vi "_create_attribute_error.vi"(1 "Is Warning (False)":bool, 4 "Original error splitter (\"Original error:\")":string="\nOriginal error:\n", 5 "Error Elaboration (\"\")":string, 6 "Error creation enabled (T)":bool=TRUE, 7 "Attribute":T2={"Identifier"="", "Descriptive Name"="", "Data Type"=enum."Integer 32", "Command"="", "Access"=enum."Read/Write", "Range Table"="", "Read Callback"="", "Write Callback"="", "Supported Models"="", "Instrument Options"="", "Index"=0, "OPC Wait"=FALSE, "No Status Check"=FALSE, "Cache Only"=FALSE}, 8 "error in":errorcluster caption="error in (no error)", 9 "Additional detail from error source (\"\")":string, 10 "Error Enum in":T1=enum."VISA_err_Timeout", 11 "VISA resource name":refnum<visa-resource-name>) -> (0 "error out":errorcluster, 3 "VISA resource name out":refnum<visa-resource-name>)   [LabVIEW 2022 SP3, in "hmp4000_rsidr_core.lvlib"]
uses:
  hmp4000_rsidr_core.lvlib
  type_Attribute.ctl
  type_Attribute_Data_Type.ctl
  type_ReadWriteAccess.ctl
  type_Error_Codes.ctl
  Trim Whitespace One-Sided.vi
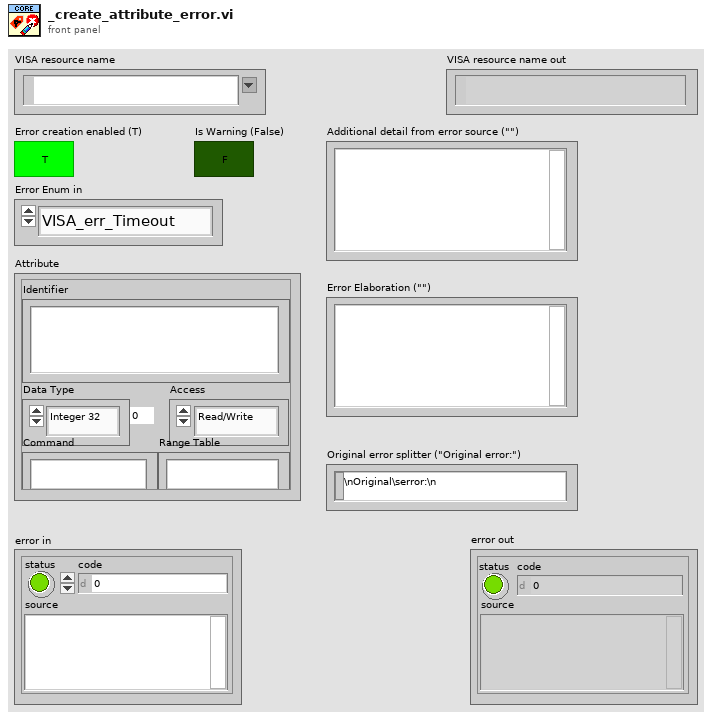
[diagram p1: front panel]
types:
  T1 = typedef "hmp4000_rsidr_core.lvlib/type_Error_Codes.ctl" = enum16{"No_error", "VISA_err_ResourceNotFound", "VISA_err_Timeout", "VISA_warn_MoreDataAvailable", "RS_err_MissingCallback", "RS_err_InvalidAttribute", "RS_err_InvalidValue", "RS_err_UnknownResource", "RS_err_AlreadyInitialized", "RS_err_InstrumentStatus", "RS_err_BadRepCapName", "RS_err_TypesMismatch", "RS_err_ValueNotSupported", "RS_err_InvalidRngTable", "RS_err_IDqueryFail", "RS_err_UnexpResponse", "VISA_warn_ConfigNotLoaded", "RS_err_AttributeNotReadable", "RS_err_AttributeNotWritable", "RS_err_InstrumentType", "RS_err_InstrumentOption", "VISA_err_InvalidSize", "RS_err_ReliabilityIndicator", "VISA_warn_UnknownStatus", "VISA_warn_TermCharRead", "VISA_err_IO_error", "RS_err_FunctionNotSupported", "VISA_warn_QueueEmpty"}
  T2 = typedef "hmp4000_rsidr_core.lvlib/type_Attribute.ctl" = cluster{"Identifier":string, "Descriptive Name":string, "Data Type":T3, "Command":string, "Access":T4, "Range Table":string, "Read Callback":string, "Write Callback":string, "Supported Models":string, "Instrument Options":string, "Index":i32, "OPC Wait":bool, "No Status Check":bool, "Cache Only":bool}
  T3 = typedef "hmp4000_rsidr_core.lvlib/type_Attribute_Data_Type.ctl" = enum16{"Integer 32", "Double", "String", "Boolean", "None", "Integer 64", "RawString"}
  T4 = typedef "hmp4000_rsidr_core.lvlib/type_ReadWriteAccess.ctl" = enum16{"Read Only", "Write Only", "Read/Write"}
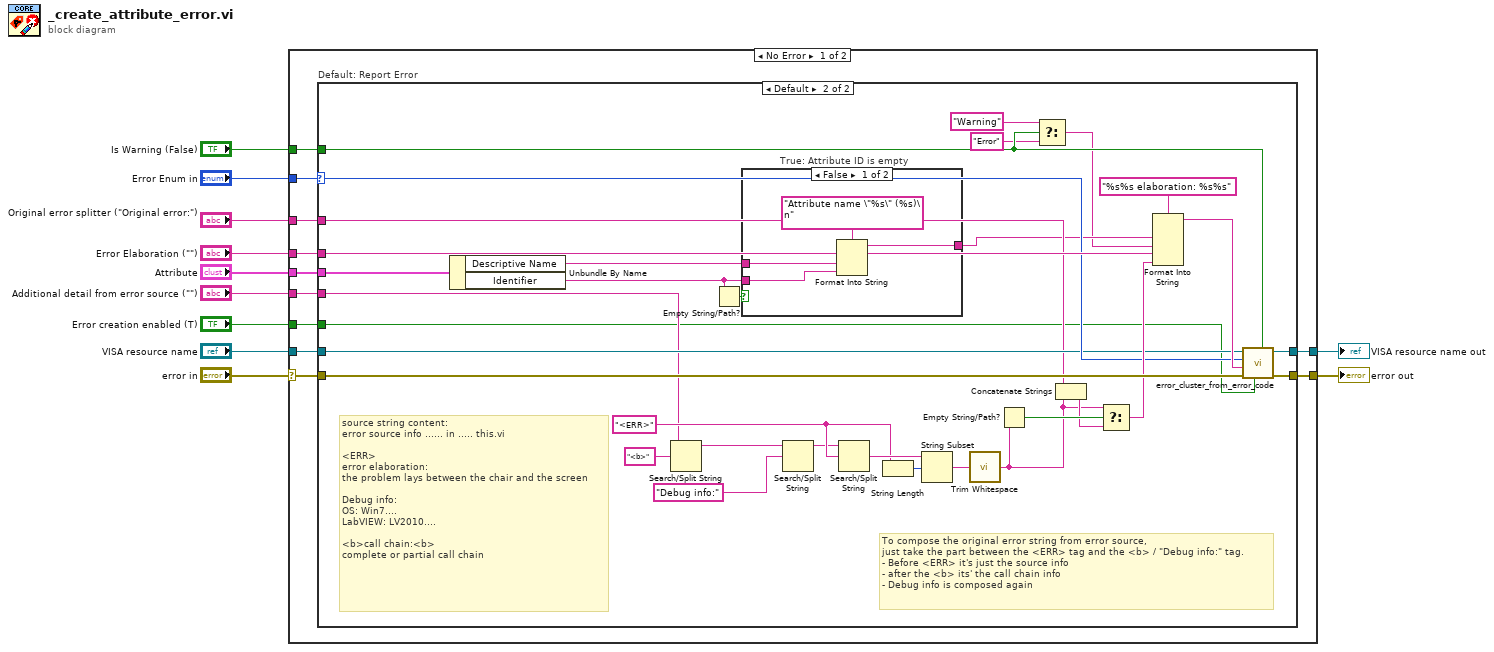
[diagram p0: block diagram]
diagram:
  n1 = case shown="No Error" "error in" {
    selector: "error in" -> [w19 w62]
    tunnel: "Attribute" -> [w20 _]
    tunnel: "Error Elaboration (\"\")" -> [w21 _]
    tunnel: [w22 w62] -> w10
    tunnel: "Error Enum in" -> [w18 _]
    tunnel: "VISA resource name" -> [w17 w61]
    tunnel: [w16 w61] -> w5
    tunnel: "Original error splitter (\"Original error:\")" -> [w15 _]
    tunnel: "Error creation enabled (T)" -> [w14 _]
    tunnel: "Additional detail from error source (\"\")" -> [w13 _]
    tunnel: "Is Warning (False)" -> [w12 _]
    frame No Error {
      n2 = case "Default: Report Error" shown="Default" w18 {
        selector: w18 -> [_ w38]
        tunnel: [w24 w53] -> w22
        tunnel: w19 -> [w24 w54]
        tunnel: w20 -> [_ w56]
        tunnel: w21 -> [_ w55]
        tunnel: w17 -> [w23 w37]
        tunnel: [w23 w36] -> w16
        tunnel: w15 -> [_ w31]
        tunnel: w14 -> [_ w30]
        tunnel: w13 -> [_ w32]
        tunnel: w12 -> [_ w28]
        frame "No_error" {
        }
        frame Default {
          w45 = "<ERR>" ("search string/char (-)")
          # "source string content:\nerror source info ...... in ..... this.vi\n\n<ERR>\nerror elaboration:\nthe problem lays between the chair and the screen\n\nDebug info:\nOS: Win7....\nLabVIEW: LV2010....\n\n<b>call chain:<b>\ncomplete or partial call chain"
          # "To compose the original error string from error source,\njust take the part between the <ERR> tag and the <b> / \"Debug info:\" tag.\n- Before <ERR> it's just the source info\n- after the <b> its' the call chain info\n- Debug info is composed again"
          n3 = Unbundle By Name(w56) -> ("Descriptive Name"=w49:string, "Identifier"=w50:string)
          n4 = Search/Split String(string=w32, search string/char (-)="<b>") -> (substring before match=w35:string)  [unwired: 1 in, 2 out]
          n5 = Empty String/Path?(string/path=w50) -> (empty?=w51:bool)
          n6 = case "True: Attribute ID is empty" shown="False" w51 {
            tunnel: w50 -> [w57 _]
            tunnel: [w59 _] -> w29
            tunnel: w49 -> [w58 _]
            frame False {
              n7 = Format Into String(format string="Attribute name \"%s\" (%s)\n", w58, w57) -> (resulting string=w59:string)  [unwired: 2 in, 1 out]
            }
            frame True {
            }
          }
          n8 = Search/Split String(string=w35, search string/char (-)="Debug info:") -> (substring before match=w33:string)  [unwired: 1 in, 2 out]
          n9 = Search/Split String(string=w33, search string/char (-)=w45) -> (match + rest of string=w47:string)  [unwired: 1 in, 2 out]
          n10 = String Length(string=w45) -> (length=w46:i32)
          n11 = String Subset(string=w47, offset (0)=w46) -> (substring=w44:string)  [unwired: 1 in]
          n12 = call "Trim Whitespace.vi"("string"=w44) -> ("trimmed string"=w40:string)  [unwired: 1 in]
          n13 = Empty String/Path?(string/path=w40) -> (empty?=w43:bool)
          n14 = Select(t="Warning", s=w28, f="Error") -> (s? t:f=w25:string)
          n15 = Concatenate Strings(w31, w40) -> (w41:string)
          n16 = Select(t=w40, s=w43, f=w41) -> (s? t:f=w42:string)
          n17 = Format Into String(format string="%s%s elaboration: %s%s", w29, w25, w55, w42) -> (resulting string=w39:string)  [unwired: 2 in, 1 out]
          n18 = call "error_cluster_from_error_code.vi"("Is Warning (False)"=w28, "Error Creation Enabled (True)"=w30, "error in"=w54, "Error Message (\"\")"=w39, "Error Enum in"=w38, "VISA resource name"=w37) -> ("error out"=w53:errorcluster, "VISA resource name out"=w36:refnum<visa-resource-name>)  [unwired: 4 in]
        }
      }
    }
    frame Error {
    }
  }
  "error out" <- w10
  "VISA resource name out" <- w5
